vi "getBoundsRect.vi"(6 "ignoreCaption&Labels":bool, 8 "error in (no error)":errorcluster, 11 "ref":refnum<vi>) -> (0 "error out":errorcluster, 2 "rect":T1, 3 "ref(dup)":refnum<vi>)   [LabVIEW 2023, in "TLC_Geometry.lvlib"]
doc: "Returns the coordinates of all the side of the object including any visible caption and label."
uses:
  TLC_Geometry.lvlib
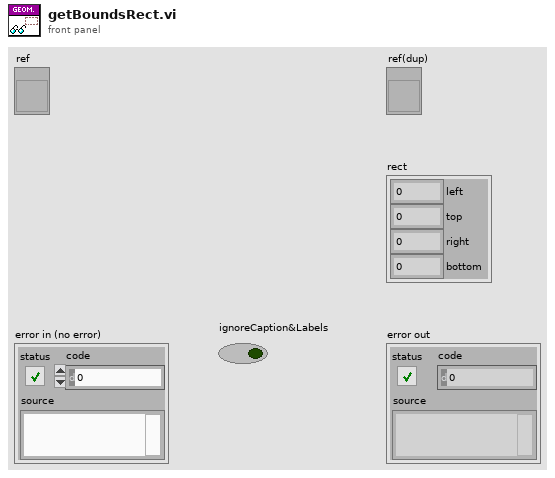
[diagram p1: front panel]
types:
  T1 = cluster{"left":i32, "top":i32, "right":i32, "bottom":i32}
  T2 = typedef "LVPositionTypeDef.ctl" = cluster{"Left":i32, "Top":i32}
  T3 = typedef "LVBoundsTypeDef.ctl" = cluster{"Width":u32, "Height":u32}
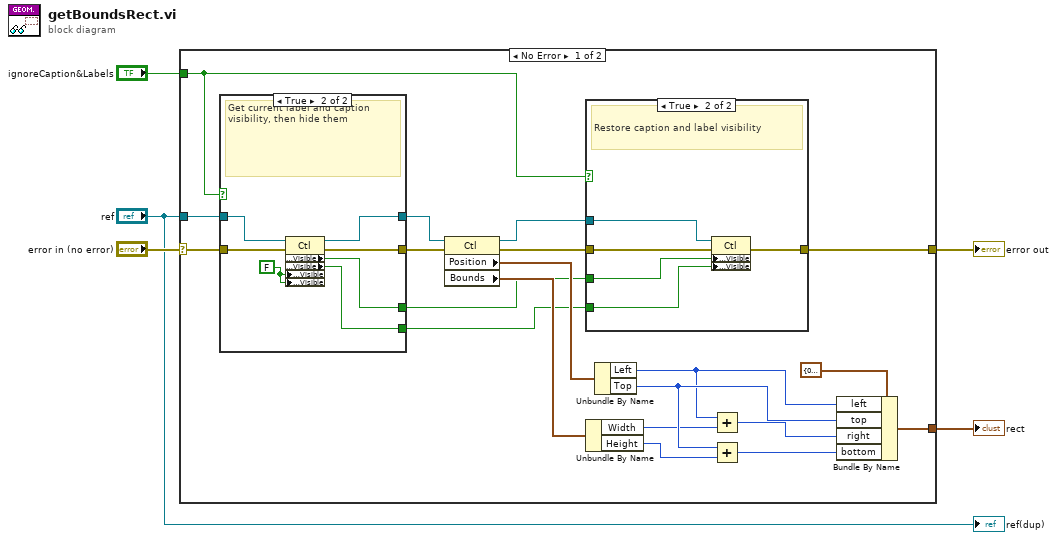
[diagram p0: block diagram]
diagram:
  n1 = case shown="No Error" "error in (no error)" {
    selector: "error in (no error)" -> [w15 w41]
    tunnel: [w25 _] -> w5
    tunnel: [w9 w41] -> w4
    tunnel: "ref" -> [w6 _]
    tunnel: "ignoreCaption&Labels" -> [w8 _]
    frame No Error {
      n2 = case shown="True" w8 {
        tunnel: [w33 w40] -> w7
        tunnel: w6 -> [w33 w39]
        tunnel: w15 -> [w32 w38]
        tunnel: [w32 w37] -> w14
        tunnel: [_ w36] -> w12
        tunnel: [_ w35] -> w11
        frame False {
          # "Do nothing"
        }
        frame True {
          w34 = FALSE ("Caption.Visible")
          # "Get current label and caption visibility, then hide them"
          n3 = property class="Ctl"(reference=w39, error in=w38, "Caption.Visible"=w34, "Label.Visible"=w34) -> (reference out=w40:refnum<vi>, error out=w37:errorcluster, "Caption.Visible"=w36:bool, "Label.Visible"=w35:bool)
        }
      }
      n4 = property class="Ctl"(reference=w7, error in=w14) -> (reference out=w13:refnum<vi>, error out=w10:errorcluster, "Position"=w17:T2, "Bounds"=w18:T3)
      n5 = case shown="True" w8 {
        tunnel: w13 -> [_ w31]
        tunnel: [w26 w30] -> w9
        tunnel: w12 -> [_ w29]
        tunnel: w11 -> [_ w28]
        tunnel: w10 -> [w26 w27]
        frame False {
          # "Do nothing"
        }
        frame True {
          # "Restore caption and label visibility"
          n6 = property class="Ctl"(reference=w31, error in=w27, "Caption.Visible"=w29, "Label.Visible"=w28) -> (error out=w30:errorcluster)  [unwired: 1 out]
        }
      }
      n7 = Unbundle By Name(w18) -> ("Width"=w20:u32, "Height"=w23:u32)
      n8 = Unbundle By Name(w17) -> ("Left"=w19:i32, "Top"=w22:i32)
      n9 = Add(x=w19, y=w20) -> (x+y=w21:u32)
      n10 = Add(x=w22, y=w23) -> (x+y=w24:u32)
      n11 = Bundle By Name(cluster=T1 {"left"=0, "top"=0, "right"=0, "bottom"=0} ("rect"), "left"=w19, "top"=w22, "right"=w21, "bottom"=w24) -> (w25:T1)
    }
    frame Error {
    }
  }
  "rect" <- w5
  "error out" <- w4
  "ref(dup)" <- "ref"
